vi "ReadXML.vi"(2 "Reinit":bool, 3 "File Path (.xml)":path) -> (0 "File Open Error":errorcluster, 1 "Data":dbl[](array[numeric]))   [LabVIEW 2019]
uses:
  <vilib>/Utility/xml.llb/Read From XML File(array).vi
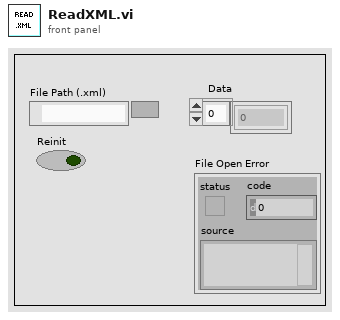
[diagram p1: front panel]
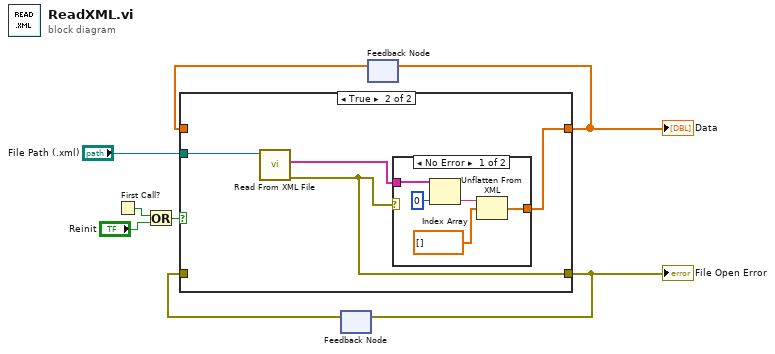
[diagram p0: block diagram]
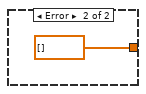
[diagram p3: hidden frame]
diagram:
  n1 = First Call?() -> (First Call?: T/F=w4:bool)
  n2 = Or(x=w4, y="Reinit") -> (x .or. y?=w5:bool)
  n3 = feedback #1() -> (w1:errorcluster)  [unwired: 1 in]
  n4 = feedback #2() -> (w6:dbl[])  [unwired: 1 in]
  n5 = case shown="True" w5 {
    tunnel: "File Path (.xml)" -> [_ w14]
    tunnel: [w10 w12] -> w7
    tunnel: w6 -> [w10 _]
    tunnel: [w9 w11] -> w2
    tunnel: w1 -> [w9 _]
    frame False {
    }
    frame True {
      n6 = call-poly <vilib>:"Read From XML File.vi"("XML File Path"=w14) -> ("error out"=w11:errorcluster, "XML Elements"=w13:string[])  [unwired: 8 in, 1 out]
      n7 = case shown="No Error" w11 {
        tunnel: w13 -> [w18 _]
        tunnel: [w16 dbl[] [] ("appended array")] -> w12
        frame No Error {
          n8 = Index Array(array=w18, index=0) -> (element=w17:string)
          n9 = Unflatten From XML(xml string=w17, type=dbl[] [] ("appended array")) -> (value=w16:dbl[])  [unwired: 1 in, 1 out]
        }
        frame Error {
        }
      }
    }
  }
  "Data" <- w7
  "File Open Error" <- w2
  n10 = feedback-in #1(w2) -> ()
  n11 = feedback-in #2(w7) -> ()
